vi "Read ADCs.vi"() -> ()   [LabVIEW 2020, in "CTI-Scratchpad.lvlib"]
uses:
  CTI-Scratchpad.lvlib
  CTI/Error Reporting.ctl
  CTI/ADC Number.ctl
  CTI/Session/Session.lvclass
  CTI/VisaComms/VisaComms.lvclass
  CTI/CTI.lvlib
panel:
  in  "Error Checking (Full)":T1=enum."Full"
  in  "Speed":i32(slide)=101 scale=1000.0..1.0
  in  "stop":bool
  out "ADC":u16[][](graph)
  in  "Port":refnum<visa-resource-name>="COM3"
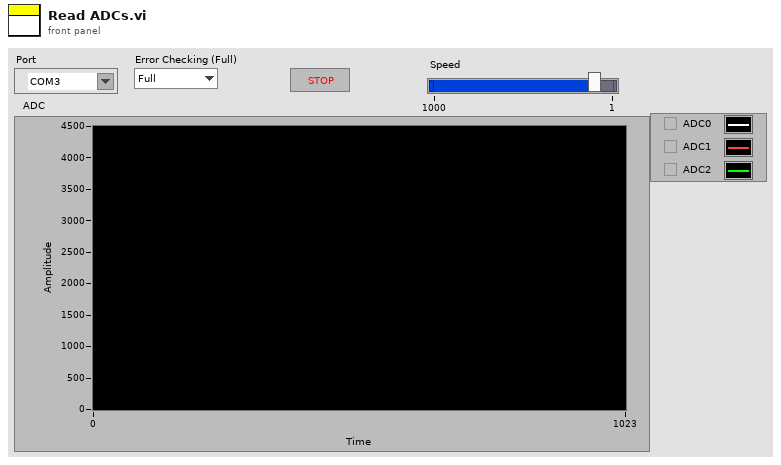
[diagram p1: front panel]
types:
  T1 = typedef "CTI.lvlib/Error Reporting.ctl" = enum16{"Minimal", "Moderate", "Full"}
  T2 = typedef "CTI.lvlib/ADC Number.ctl" = i8
  T3 = typedef "CTI.lvlib/Raw ADC.ctl" = u16
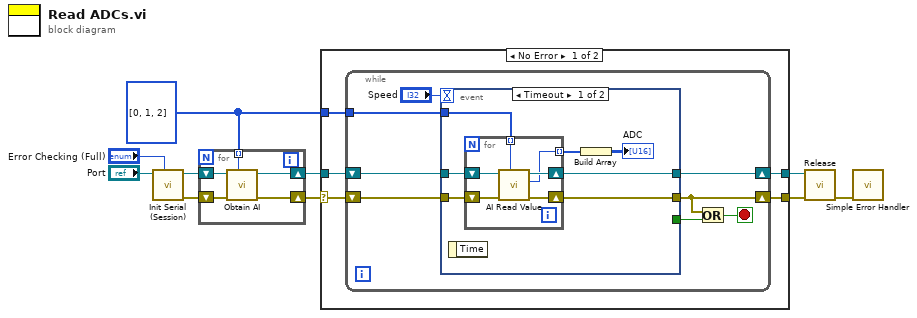
[diagram p0: block diagram]
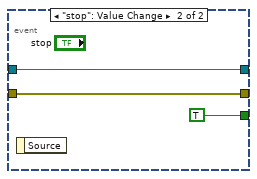
[diagram p2: hidden frame]
diagram:
  w2 = T2[] [0, 1, 2]
  n1 = call "Init Serial (Session).vi"("Error Checking (Full)"="Error Checking (Full)", "VISA resource name in"="Port") -> ("error out"=w8:errorcluster, "Session"=w9:refnum<class "Session.lvclass">)  [unwired: 7 in, 1 out]
  n2 = for {
    shift-right: [w13] -> w6
    shift-left: w9 -> [w15]
    shift-right: [w12] -> w7
    shift-left: w8 -> [w14]
    tunnel: w2 -> [w11] mode=indexing
    n3 = call "Obtain AI.vi"("ADC #"=w11, "error in (no error)"=w14, "Session in"=w15) -> ("error out"=w12:errorcluster, "Session out"=w13:refnum<class "Session.lvclass">)  [unwired: 7 in]
  }
  n4 = case shown="No Error" w7 {
    selector: w7 -> [w18 w46]
    tunnel: w6 -> [w19 w45]
    tunnel: w2 -> [w20 _]
    tunnel: [w16 w46] -> w4
    tunnel: [w17 w45] -> w5
    frame No Error {
      n5 = while {
        tunnel: w20 -> [w27]
        shift-right: [w24] -> w17
        shift-left: w19 -> [w26]
        shift-right: [w23] -> w16
        shift-left: w18 -> [w25]
        stop <- w21 stop-if-true
        n6 = event shown="[0] Timeout" {
          selector: _ -> [_ _]
          dyn-events: _ -> [_ _]
          timeout: "Speed" -> [_ _]
          tunnel: w27 -> [w33 _]
          tunnel: w26 -> [w35 w42]
          tunnel: w25 -> [w34 w43]
          tunnel: [w30 w42] -> w24
          tunnel: [w29 w43] -> w23
          tunnel: [_ TRUE] -> w22
          event Timeout {
            n7 = event-data() -> ()  [unwired: 1 in, 1 out]
            n8 = for {
              shift-right: [w39] -> w30
              shift-left: w35 -> [w41]
              shift-right: [w38] -> w29
              shift-left: w34 -> [w40]
              tunnel: w33 -> [w36] mode=indexing
              tunnel: [w37] -> w31 mode=indexing
              n9 = call "AI Read Value.vi"("ADC #"=w36, "error in (no error)"=w40, "Session in"=w41) -> ("error out"=w38:errorcluster, "Value"=w37:T3, "Session out"=w39:refnum<class "Session.lvclass">)  [unwired: 6 in]
            }
            n10 = Build Array(w31) -> (→"ADC":T3[][])
          }
          event "stop": Value Change {
            n11 = event-data() -> ()  [unwired: 1 in, 1 out]
          }
        }
        n12 = Or(x=w23, y=w22) -> (x .or. y?=w21:bool)
      }
    }
    frame Error {
    }
  }
  n13 = call-dynamic "Release.vi"("error in (no error)"=w4, "Session in"=w5) -> ("error out"=w3:errorcluster)  [unwired: 9 in]
  n14 = call <vilib>:"Simple Error Handler.vi"("error in (no error)"=w3) -> ()  [unwired: 4 in, 5 out]
